vi "Signal Selection.vi"(7 "Signal":T1, 8 "error in":errorcluster, 11 "DATA IN":T2) -> (0 "error out":errorcluster, 2 "Fs":u32, 3 "Display OUT":waveform(dbl))   [LabVIEW 2017, in "Processing.lvlib"]
uses:
  Processing.lvlib
  support/libs/PMU Buffer/Buffer DATA OUT ordered.ctl
  Display Select.ctl
  <vilib>/Analysis/baseanly.llb/Mean (DBL).vi
  <vilib>/Analysis/NI_AALBase.lvlib
  support/libs/PMU Buffer/PMU data buffer.lvlib
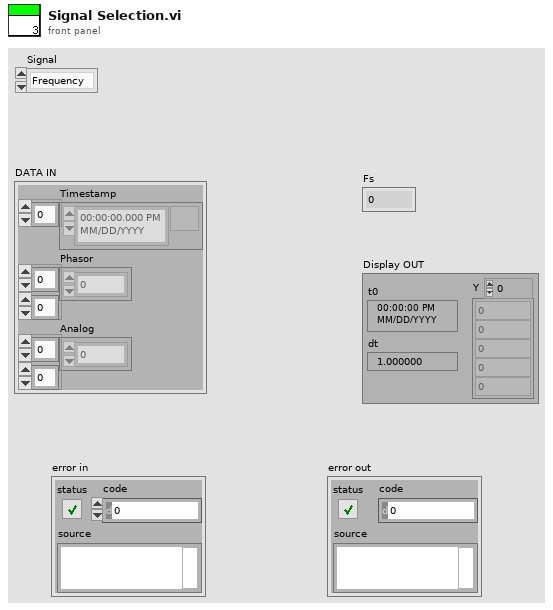
[diagram p1: front panel]
types:
  T1 = typedef "Processing.lvlib/Display Select.ctl" = enum16{"Frequency", "Voltage"}
  T2 = typedef "PMU data buffer.lvlib/Buffer DATA OUT ordered.ctl" = cluster{"Timestamp":timestamp[], "Phasor":csg[][], "Analog":sgl[][]}
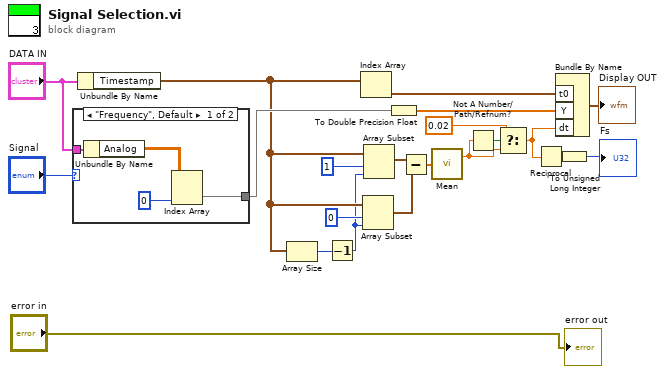
[diagram p0: block diagram]
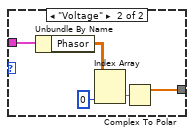
[diagram p2: hidden frame]
diagram:
  n1 = case shown="\"Frequency\", Default" "Signal" {
    tunnel: [w24 w26] -> w19
    tunnel: "DATA IN" -> [w23 w28]
    frame "Frequency", Default {
      n2 = Unbundle By Name(w23) -> ("Analog"=w22:sgl[][])
      n3 = Index Array(array=w22, index (col)=0 ("disabled index (col)")) -> (element=w24:sgl[])  [unwired: 1 in]
    }
    frame "Voltage" {
      n4 = Unbundle By Name(w28) -> ("Phasor"=w27:csg[][])
      n5 = Index Array(array=w27, index (col)=0 ("disabled index (col)")) -> (element=w30:csg[])  [unwired: 1 in]
      n6 = Complex To Polar(r * e^(i*theta)=w30) -> (r=w26:sgl[])  [unwired: 1 out]
    }
  }
  n7 = Unbundle By Name("DATA IN") -> ("Timestamp"=w12:timestamp[])
  n8 = Array Size(array=w12) -> (size(s)=w13:i32)
  n9 = Decrement(x=w13) -> (x-1=w11:i32)
  n10 = Index Array(array=w12) -> (element=w21:timestamp)  [unwired: 1 in]
  n11 = Array Subset(array=w12, index=0, length=w11) -> (w9:timestamp[])
  n12 = Array Subset(array=w12, index=1, length=w11) -> (w10:timestamp[])
  n13 = To Double Precision Float(number=w19) -> (double precision float=w5:dbl[])
  n14 = Subtract(x=w10, y=w9) -> (x-y=w8:dbl[])
  n15 = call-poly <vilib>:"Mean.vi"("X"=w8) -> ("mean"=w2:dbl)  [unwired: 1 out]
  n16 = Not A Number/Path/Refnum?(number/path/refnum=w2) -> (NaN/Path/Refnum?=w4:bool)
  n17 = Select(t=0.02, s=w4, f=w2) -> (s? t:f=w3:dbl)
  n18 = Reciprocal(x=w3) -> (1/x=w7:dbl)
  n19 = Bundle By Name("t0"=w21, "Y"=w5, "dt"=w3) -> (→"Display OUT":waveform(dbl))  [unwired: 1 in]
  n20 = To Unsigned Long Integer(number=w7) -> (unsigned 32bit integer=→"Fs":u32)
  "error out" <- "error in"
